vi "setState.vi"(8 "error in (no error)":errorcluster, 10 "state":bool, 11 "Pump in":refnum<class "Pump.lvclass">) -> (0 "error out":errorcluster, 3 "Pump out":refnum<class "Pump.lvclass">)   [LabVIEW 2018, in "Pump.lvclass"]
uses:
  Pump.lvclass
  Pump.lvclass/Pump.ctl
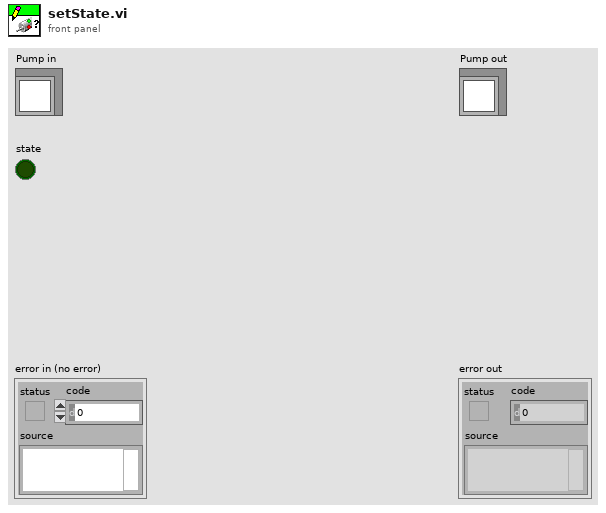
[diagram p1: front panel]
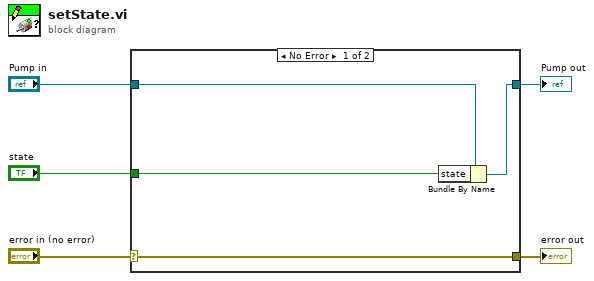
[diagram p0: block diagram]
diagram:
  n1 = case shown="No Error" "error in (no error)" {
    selector: "error in (no error)" -> [w9 w10]
    tunnel: [w9 w10] -> w4
    tunnel: [w7 w11] -> w2
    tunnel: "Pump in" -> [w8 w11]
    tunnel: "state" -> [w6 _]
    frame No Error {
      n2 = Bundle By Name(cluster=w8, "state"=w6) -> (w7:refnum<class "Pump.lvclass">)
    }
    frame Error {
    }
  }
  "error out" <- w4
  "Pump out" <- w2
